vi "Create.vi"(8 "error in (no error)":errorcluster caption="错误输入（无错误）", 11 "User Event Collection 输入":refnum<class "User Event Collection.lvclass"> caption="DNL_LabVIEW Object in") -> (0 "error out":errorcluster caption="错误输出", 3 "User Event Collection 输出":refnum<class "User Event Collection.lvclass"> caption="DNL_LabVIEW Object out")   [LabVIEW 2013, in "User Event Collection.lvclass"]
uses:
  User Event Collection.lvclass
  Tag.ctl
  <resource>/importtools/Common/Event/NISAST Event.lvclass
  User Event Collection.lvclass/User Event Collection.ctl
panel:
  in  "Tag":T1
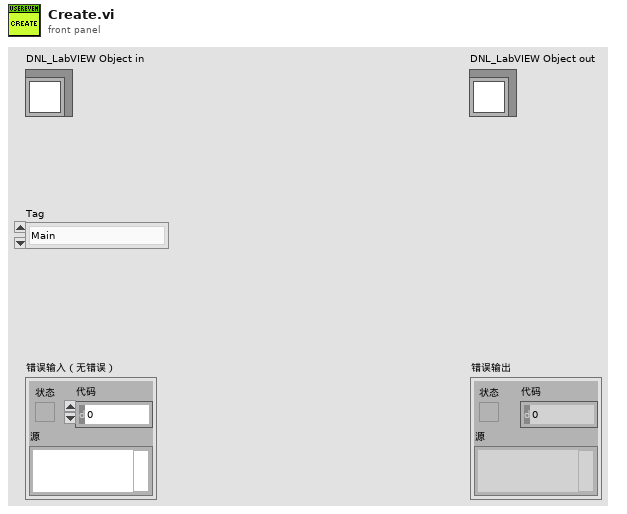
[diagram p1: front panel]
types:
  T1 = typedef "User Event Collection.lvclass/Tag.ctl" = enum16{"Main", "UI"}
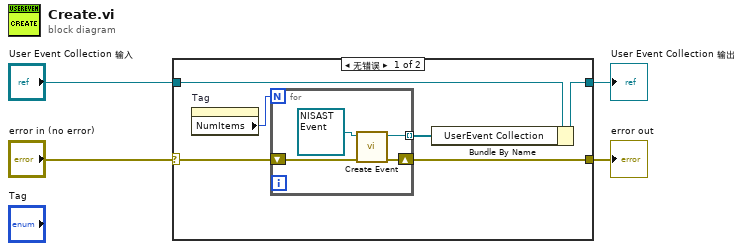
[diagram p0: block diagram]
diagram:
  n1 = case shown="无错误" "error in (no error)" {
    selector: "error in (no error)" -> [w7 w16]
    tunnel: [w6 w16] -> w3
    tunnel: [w9 w15] -> w1
    tunnel: "User Event Collection 输入" -> [w10 w15]
    frame No Error {
      n2 = property on="Tag" class="Enum (严格)"() -> ("NumItems"=w5:u32)  [unwired: 2 in, 2 out]
      n3 = for {
        N: w5 -> [_]
        tunnel: [w14] -> w8 mode=indexing
        shift-right: [w11] -> w6
        shift-left: w7 -> [w12]
        n4 = call-dynamic "Create Event.vi"("error in (no error)"=w12, "Event in"=refnum<class "NISAST Event.lvclass"> refnum) -> ("error out"=w11:errorcluster, "Event out"=w14:refnum<class "NISAST Event.lvclass">)  [unwired: 7 in, 1 out]
      }
      n5 = Bundle By Name(cluster=w10, "UserEvent Collection"=w8) -> (w9:refnum<class "User Event Collection.lvclass">)
    }
    frame Error {
    }
  }
  "error out" <- w3
  "User Event Collection 输出" <- w1
